vi "main.vi"() -> ()   [LabVIEW 2021]
uses:
  states_enum_typedef.ctl
  data_cluster_typedef.ctl
  <vilib>/Utility/file.llb/Write Delimited Spreadsheet (DBL).vi
  <vilib>/Instr/_visa.llb/VISA Configure Serial Port (Instr).vi
  <vilib>/Utility/file.llb/Read Delimited Spreadsheet (DBL).vi
panel:
  out "error out":errorcluster
  out "State":T1
  out "Time Displacement":cluster{"Time":dbl[], "Displacement":dbl[]}(graph)
  out "Time Stress":cluster{"Time":dbl[], "Load":dbl[]}(graph)
  out "Stress Displacement":cluster{"Load":dbl[], "Displacement":dbl[]}(graph)
  out "Connected?":bool
  in  "Serial Port":refnum<visa-resource-name>
  in  "Disconnect":bool
  in  "Connect":bool
  in  "Clear":bool
  in  "Save":bool
  in  "Load":bool
  in  "Exit":bool
  # "Spring Slider Earthquake Machine"
  # "1) Connect your stick-slip machine to the computer\n2) Select the appropriate serial port from the list\n3) Click \"Connect\"\n4) Run your experiment\n5) Save the data if desired, then clear the chart\n6) When all experiments are done, click \"Disconnect\""
  # "V1.1"
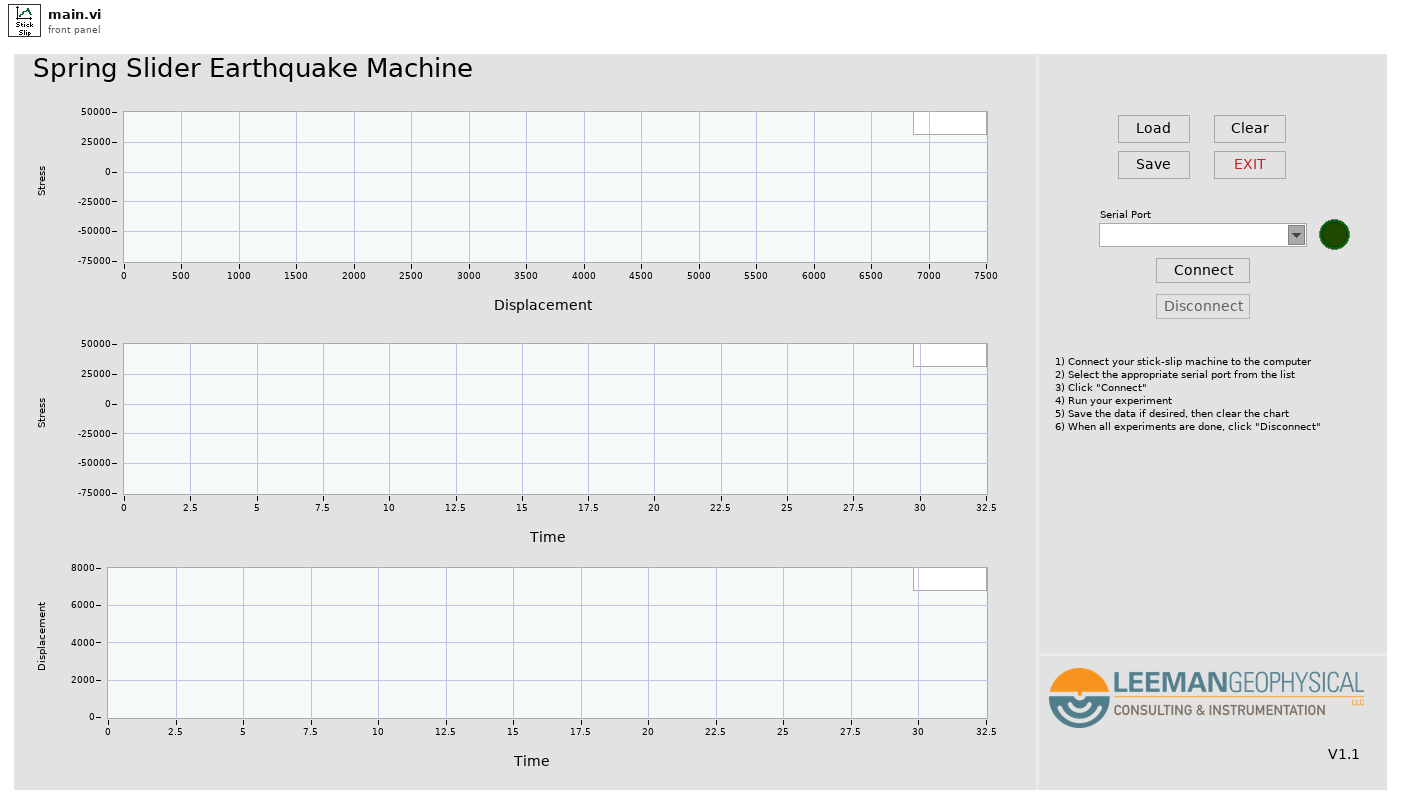
[diagram p1: front panel]
types:
  T1 = typedef "states_enum_typedef.ctl" = enum16{"Shutdown", "Update", "Initialize", "Clear", "Save", "Connect", "Disconnect", "Load", "Wait"}
  T2 = enum8{"Enabled", "Disabled", "Disabled and Grayed Out"}
  T3 = typedef "data_cluster_typedef.ctl" = cluster{"Time":dbl[], "Displacement":dbl[], "Load":dbl[]}
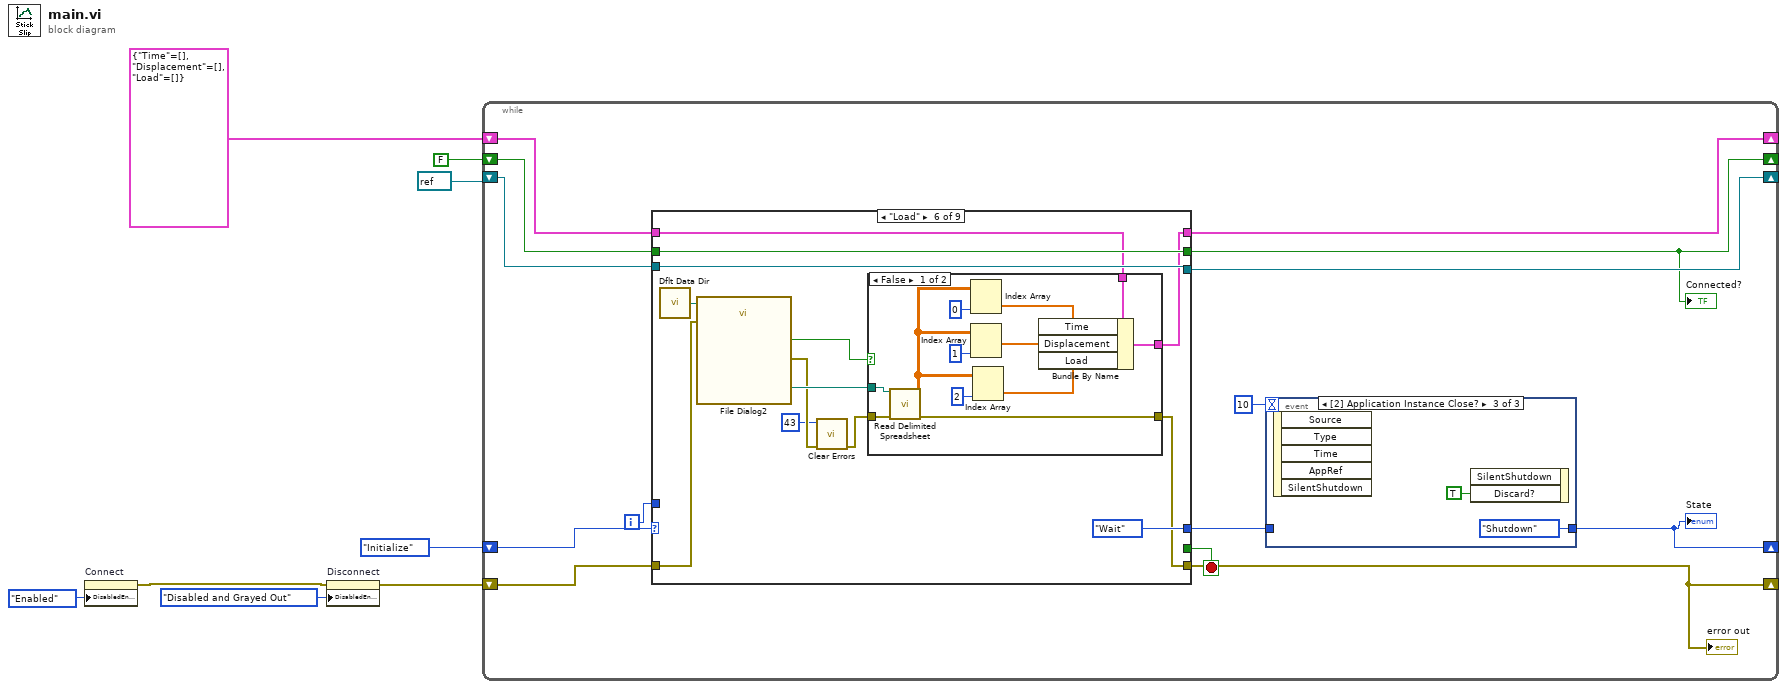
[diagram p0: block diagram]
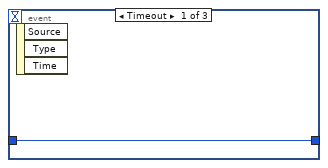
[diagram p2: hidden frame]
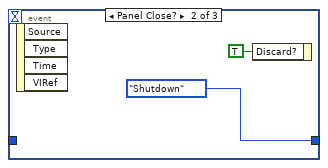
[diagram p3: hidden frame]
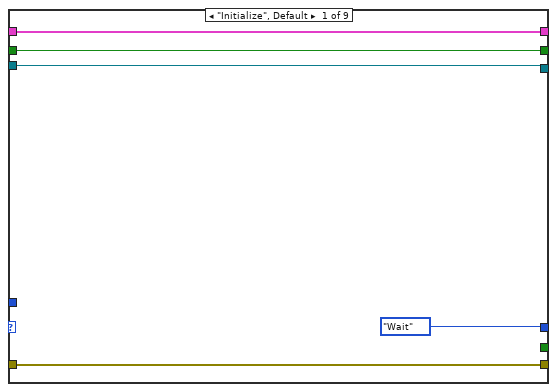
[diagram p4: hidden frame]
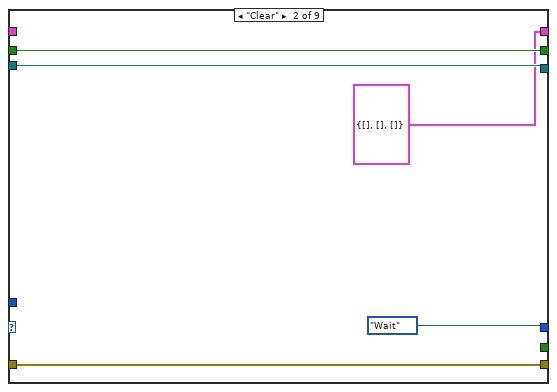
[diagram p5: hidden frame]
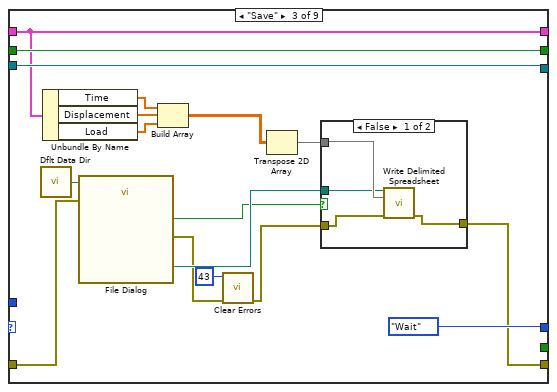
[diagram p6: hidden frame]
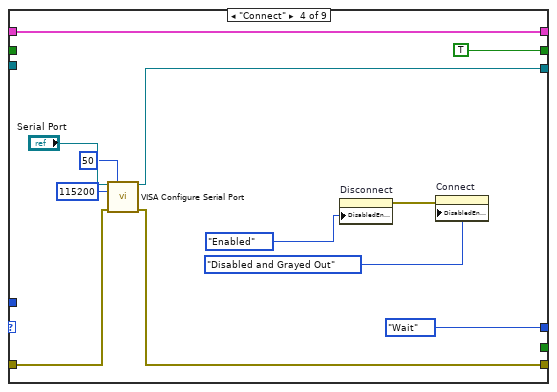
[diagram p8: hidden frame]
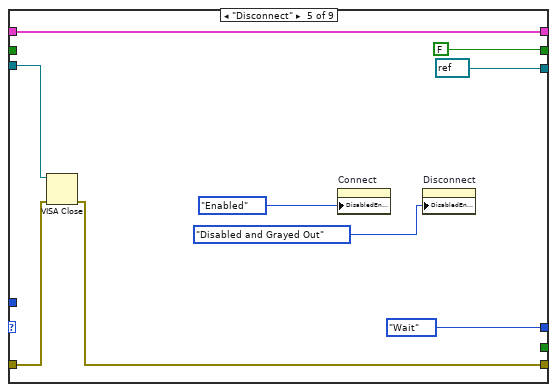
[diagram p9: hidden frame]
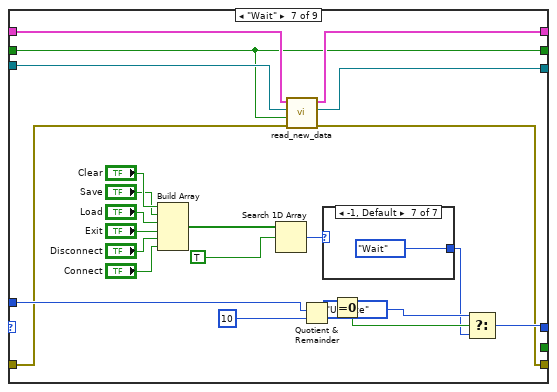
[diagram p11: hidden frame]
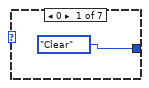
[diagram p12: hidden frame]
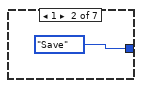
[diagram p13: hidden frame]
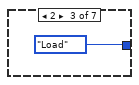
[diagram p14: hidden frame]
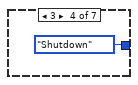
[diagram p15: hidden frame]
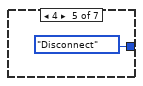
[diagram p16: hidden frame]
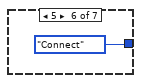
[diagram p17: hidden frame]
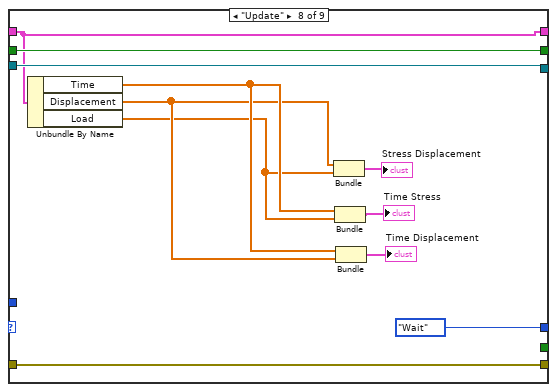
[diagram p18: hidden frame]
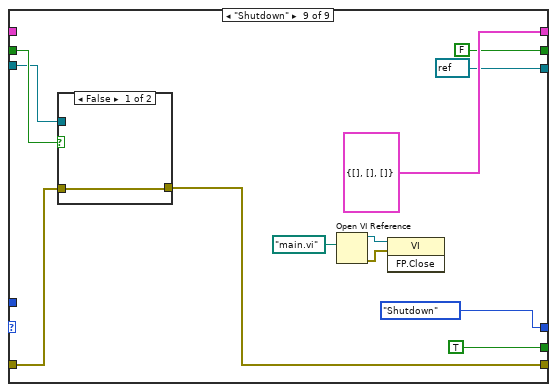
[diagram p19: hidden frame]
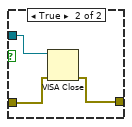
[diagram p20: hidden frame]
diagram:
  n1 = property on="Connect" class="Bool"("DisabledEnum"=T2."Enabled" ("Disabled")) -> (error out=w2:errorcluster)  [unwired: 2 in, 1 out]
  n2 = property on="Disconnect" class="Bool"(error in=w2, "DisabledEnum"=T2."Disabled and Grayed Out" ("Disabled")) -> (error out=w1:errorcluster)  [unwired: 1 in, 1 out]
  n3 = while {
    shift-right: [w11] -> _
    shift-left: states_enum_typedef."Initialize" -> [w22]
    shift-right: [w15] -> _
    shift-left: T3 {"Time"=[], "Displacement"=[], "Load"=[]} -> [w20]
    shift-right: [w12] -> _
    shift-left: FALSE -> [w21]
    shift-right: [w18] -> _
    shift-left: w1 -> [w19]
    shift-right: [w17] -> _
    shift-left: refnum<visa-resource-name> refnum ("VISA resource name out") -> [w16]
    i -> [w14]
    stop <- w13 stop-if-true
    n4 = case shown="\"Load\"" w22 {
      tunnel: w21 -> [w31 w37 w54 _ _ w93 w110 w148 w159]
      tunnel: w20 -> [w32 _ w51 w66 w76 w89 w114 w144 _]
      tunnel: w19 -> [w29 w34 w38 w69 w78 w81 w109 w146 w157]
      tunnel: [w29 w34 w42 w60 w72 w90 w108 w146 w156] -> w18
      tunnel: [w30 w36 w53 w68 refnum<visa-resource-name> refnum ("VISA resource name out") w92 w111 w147 refnum<visa-resource-name> refnum ("VISA resource name out")] -> w17
      tunnel: w16 -> [w30 w36 w53 _ w80 w92 w112 w147 w158]
      tunnel: [w31 w37 w54 TRUE FALSE w93 w110 w148 FALSE] -> w12
      tunnel: [w32 T3 {"Time"=[], "Displacement"=[], "Load"=[]} w51 w66 w76 w88 w113 w144 T3 {"Time"=[], "Displacement"=[], "Load"=[]}] -> w15
      tunnel: [states_enum_typedef."Wait" states_enum_typedef."Wait" states_enum_typedef."Wait" states_enum_typedef."Wait" states_enum_typedef."Wait" states_enum_typedef."Wait" w119 states_enum_typedef."Wait" states_enum_typedef."Shutdown"] -> w10
      tunnel: w14 -> [_ _ _ _ _ _ w123 _ _]
      tunnel: [_ _ _ _ _ _ _ _ TRUE] -> w13
      frame "Initialize", Default {
      }
      frame "Clear" {
      }
      frame "Save" {
        n5 = call <vilib>:"Dflt Data Dir.vi"() -> ("App:Default Data Directory"=w44:path)
        n6 = Unbundle By Name(w51) -> ("Time"=w50:dbl[], "Displacement"=w49:dbl[], "Load"=w48:dbl[])
        n7 = call "File Dialog"("start path"=w44, "error in"=w38) -> ("selected path"=w45:path, "cancelled"=w43:bool, "error out"=w41:errorcluster)  [unwired: 10 in, 1 out]
        n8 = Build Array(w50, w49, w48) -> (w47:dbl[][])
        n9 = call <vilib>:"Clear Errors.vi"("error in (no error)"=w41, "specific error code to clear (0: all)"=43) -> ("error out"=w39:errorcluster)  [unwired: 4 in, 1 out]
        n10 = Transpose 2D Array(2D array=w47) -> (transposed array=w46:dbl[][])
        n11 = case shown="False" w43 {
          tunnel: w39 -> [w56 w59]
          tunnel: w46 -> [w58 _]
          tunnel: w45 -> [w57 _]
          tunnel: [w55 w59] -> w42
          frame False {
            n12 = call-poly <vilib>:"Write Delimited Spreadsheet.vi"("file path (dialog if empty)"=w57, "2D data"=w58, "error in (no error)"=w56) -> ("error out"=w55:errorcluster)  [unwired: 11 in, 1 out]
          }
          frame True {
          }
        }
      }
      frame "Connect" {
        n13 = call-poly "VISA Configure Serial Port"("VISA resource name"="Serial Port", "timeout (10sec)"=u32 50, "baud rate (9600)"=u32 115200, "error in (no error)"=w69) -> ("VISA resource name out"=w68:refnum<visa-resource-name>, "error out"=w60:errorcluster)  [unwired: 10 in]
        n14 = property on="Disconnect" class="Bool"("DisabledEnum"=T2."Enabled" ("Disabled")) -> (error out=w62:errorcluster)  [unwired: 2 in, 1 out]
        n15 = property on="Connect" class="Bool"(error in=w62, "DisabledEnum"=T2."Disabled and Grayed Out" ("Disabled")) -> ()  [unwired: 1 in, 2 out]
      }
      frame "Disconnect" {
        n16 = VISA Close(VISA resource name=w80, error in (no error)=w78) -> (error out=w72:errorcluster)
        n17 = property on="Connect" class="Bool"("DisabledEnum"=T2."Enabled" ("Disabled")) -> ()  [unwired: 2 in, 2 out]
        n18 = property on="Disconnect" class="Bool"("DisabledEnum"=T2."Disabled and Grayed Out" ("Disabled")) -> ()  [unwired: 2 in, 2 out]
      }
      frame "Load" {
        n19 = call <vilib>:"Dflt Data Dir.vi"() -> ("App:Default Data Directory"=w87:path)
        n20 = call "File Dialog2"("start path"=w87, "error in"=w81) -> ("selected path"=w86:path, "cancelled"=w85:bool, "error out"=w84:errorcluster)  [unwired: 10 in, 1 out]
        n21 = call <vilib>:"Clear Errors.vi"("error in (no error)"=w84, "specific error code to clear (0: all)"=43) -> ("error out"=w82:errorcluster)  [unwired: 4 in, 1 out]
        n22 = case shown="False" w85 {
          tunnel: [w105 w106] -> w90
          tunnel: w89 -> [w100 w107]
          tunnel: [w96 w107] -> w88
          tunnel: w86 -> [w95 _]
          tunnel: w82 -> [w94 w106]
          frame False {
            n23 = call-poly <vilib>:"Read Delimited Spreadsheet.vi"("file path (dialog if empty)"=w95, "error in (no error)"=w94) -> ("all rows"=w101:dbl[][], "error out"=w105:errorcluster)  [unwired: 8 in, 4 out]
            n24 = Index Array(array=w101, index (col)=0 ("disabled index (col)")) -> (element=w99:dbl[])  [unwired: 1 in]
            n25 = Index Array(array=w101, index (col)=1 ("disabled index (col)")) -> (element=w98:dbl[])  [unwired: 1 in]
            n26 = Index Array(array=w101, index (col)=2 ("disabled index (col)")) -> (element=w97:dbl[])  [unwired: 1 in]
            n27 = Bundle By Name(cluster=w100, "Time"=w99, "Displacement"=w98, "Load"=w97) -> (w96:T3)
          }
          frame True {
          }
        }
      }
      frame "Wait" {
        n28 = Build Array("Clear", "Save", "Load", "Exit", "Disconnect", "Connect") -> (w118:bool[])
        n29 = Search 1D Array(1D array=w118, element=TRUE) -> (index of element=w116:i32)  [unwired: 1 in]
        n30 = call "read_new_data.vi"("Error In"=w109, "connected?"=w110, "VISA in"=w112, "Data Cluster In"=w114) -> ("Error Out"=w108:errorcluster, "VISA out"=w111:refnum<visa-resource-name>, "Data Cluster Out"=w113:T3)  [unwired: 5 in]
        n31 = Quotient & Remainder(x=w123, y=10) -> (x-y*floor(x/y)=w122:i32)  [unwired: 1 out]
        n32 = case shown="-1, Default" w116 {
          tunnel: [states_enum_typedef."Clear" states_enum_typedef."Save" states_enum_typedef."Load" states_enum_typedef."Shutdown" states_enum_typedef."Disconnect" states_enum_typedef."Connect" states_enum_typedef."Wait"] -> w115
          frame 0 {
          }
          frame 1 {
          }
          frame 2 {
          }
          frame 3 {
          }
          frame 4 {
          }
          frame 5 {
          }
          frame -1, Default {
          }
        }
        n33 = Equal To 0?(x=w122) -> (x = 0?=w121:bool)
        n34 = Select(t=states_enum_typedef."Update", s=w121, f=w115) -> (s? t:f=w119:T1)
      }
      frame "Update" {
        n35 = Unbundle By Name(w144) -> ("Time"=w141:dbl[], "Displacement"=w139:dbl[], "Load"=w138:dbl[])
        n36 = Bundle("Displacement"=w139, "Load"=w138) -> (→"Stress Displacement":cluster{"Displacement":dbl[], "Load":dbl[]})  [unwired: 1 in]
        n37 = Bundle("Time"=w141, "Load"=w138) -> (→"Time Stress":cluster{"Time":dbl[], "Load":dbl[]})  [unwired: 1 in]
        n38 = Bundle("Time"=w141, "Displacement"=w139) -> (→"Time Displacement":cluster{"Time":dbl[], "Displacement":dbl[]})  [unwired: 1 in]
      }
      frame "Shutdown" {
        n39 = case shown="False" w159 {
          tunnel: w158 -> [_ w164]
          tunnel: w157 -> [w161 w163]
          tunnel: [w161 w162] -> w156
          frame False {
          }
          frame True {
            n40 = VISA Close(VISA resource name=w164, error in (no error)=w163) -> (error out=w162:errorcluster)
          }
        }
        n41 = Open VI Reference(vi path=path "main.vi") -> (vi reference=w150:refnum<vi>, error out=w149:errorcluster)  [unwired: 5 in]
        n42 = invoke class="VI" method="FP.Close"(reference=w150, error in=w149) -> ()  [unwired: 1 in, 3 out]
      }
    }
    "Connected?" <- w12
    "error out" <- w18
    n43 = event shown="[2] Application Instance Close?" {
      selector: _ -> [_ _ _]
      dyn-events: _ -> [_ _ _]
      timeout: 10 -> [_ _ _]
      tunnel: [w23 states_enum_typedef."Shutdown" states_enum_typedef."Shutdown"] -> w11
      tunnel: w10 -> [w23 _ _]
      event Timeout {
        n44 = event-data() -> ()  [unwired: 1 in, 3 out]
      }
      event Panel Close? {
        n45 = event-data() -> ()  [unwired: 1 in, 4 out]
        n46 = event-data("Discard?"=TRUE) -> ()  [unwired: 1 in, 1 out]
      }
      event Application Instance Close? {
        n47 = event-data() -> ()  [unwired: 1 in, 5 out]
        n48 = event-data("Discard?"=TRUE) -> ()  [unwired: 2 in, 1 out]
      }
    }
    "State" <- w11
  }
